vi "PhotonPoseEstimator_Execute.vi"(7 "Configuration":T9, 9 "ReferencePose":T4={"Translation3d"={"X"=0.0, "Y"=0.0, "Z"=0.0}, "Rotation3d"={"Q_quaternion"={"R"=1.0, "V"=[0.0, 0.0, 0.0]}}} {"Translation3d"."Z" format="%14.3f"; "Translation3d"."Y" format="%14.3f"; "Translation3d"."X" format="%14.3f"}, 10 "PIpeline Has \nNew Results":bool, 11 "PipelineResult":T10) -> (0 "TimeStamp_Seconds":dbl, 1 "New Pose Found":bool, 2 "EstimatedPose2d":T1={"TRANSLATION"={"X"=0.0, "Y"=0.0}, "ROTATION"={"VALUE"=0.0, "COS"=1.0, "SIN"=0.0}} {"ROTATION"."SIN" format="%13.4f"; "ROTATION"."COS" format="%13.4f"; "ROTATION"."VALUE" format="%13.4f"; "TRANSLATION"."Y" format="%14.3f"; "TRANSLATION"."X" format="%14.3f"}, 3 "EstimatedPose3d":T4={"Translation3d"={"X"=0.0, "Y"=0.0, "Z"=0.0}, "Rotation3d"={"Q_quaternion"={"R"=1.0, "V"=[0.0, 0.0, 0.0]}}} {"Translation3d"."Z" format="%14.3f"; "Translation3d"."Y" format="%14.3f"; "Translation3d"."X" format="%14.3f"}, 4 "Strategy Used":T8, 5 "PhotonEstimatedRobotPose":T11={"EstimatedPose"={"Translation3d"={"X"=0.0, "Y"=0.0, "Z"=0.0}, "Rotation3d"={"Q_quaternion"={"R"=1.0, "V"=[0.0, 0.0, 0.0]}}}, "TimeStamp_Seconds"=0.0, "targetsUsed"=[], "Strategy"=enum."LOWEST_AMBIGUITY"} {"targetsUsed"."AltCameraToTarget"."TRANSLATION3D"."Z" format="%14.3f"; "targetsUsed"."AltCameraToTarget"."TRANSLATION3D"."Y" format="%14.3f"; "targetsUsed"."AltCameraToTarget"."TRANSLATION3D"."X" format="%14.3f"; "targetsUsed"."BestCameraToTarget"."TRANSLATION3D"."Z" format="%14.3f"; "targetsUsed"."BestCameraToTarget"."TRANSLATION3D"."Y" format="%14.3f"; "targetsUsed"."BestCameraToTarget"."TRANSLATION3D"."X" format="%14.3f"; "EstimatedPose"."Translation3d"."Z" format="%14.3f"; "EstimatedPose"."Translation3d"."Y" format="%14.3f"; "EstimatedPose"."Translation3d"."X" format="%14.3f"}, 6 "out PhotonPoseEstimator":T15)   [LabVIEW 2019, in "PhotonVisionLib.lvlib"]
doc: "Provided data from polling a camera, update the estimated position of the robot. Returns empty if there are no cameras set or no targets were found from the cameras. \n\nInputs:\n -- PhotonPoseEstimator -- data cluster -- Data guiding how the position determination is done.\n -- PipelineResults -- data cluster -- Data provided from PhotonCamera_GetLatestResults.\n -- HasResults -- boolean - TRUE if targets have been identified in the Pipeline results. This can be provided by PhotonCamera_GetLatestResults.\n\nOutputs:\n - EstimatedPose3d - Pose3d - Estimated 3d position. Only value if NewPoseFound = TRUE\n - EstimatedPose2d - Pose2d - Estimated 2d position. Only value if NewPoseFound = TRUE\n - NewPoseFound -- boolean -- A new position has been determined.\n - TimeStampe - double - Target timestamp (seconds)\n - StrategyUsed -- enum -- The strategy used to determine the pose.\n - PhotonEstimatedRobotPose -- data cluster -- Complete estimated robot position and timestamp data cluster\n -- PhotonPoseEstimator -- data cluster -- Updated data cluster."
uses:
  PhotonVisionLib.lvlib
  Ref/PhotonPoseEstimator_REF.ctl
  TypeDef/PhotonPoseEstimatorType.ctl
  <vilib>/Rock Robotics/WPI/ThirdParty/JAS_Junk/TrajLib/TypeDef/POSE3D.ctl
  <vilib>/Rock Robotics/WPI/ThirdParty/JAS_Junk/TrajLib/TypeDef/TRANSLATION3D.ctl
  <vilib>/Rock Robotics/WPI/ThirdParty/JAS_Junk/TrajLib/TypeDef/ROTATION3D.ctl
  <vilib>/Rock Robotics/WPI/ThirdParty/JAS_Junk/TrajLib/TypeDef/QUATERNION.ctl
  <vilib>/Rock Robotics/WPI/ThirdParty/JAS_Junk/TrajLib/TypeDef/AprilTagFieldLayout.ctl
  <vilib>/Rock Robotics/WPI/ThirdParty/JAS_Junk/TrajLib/TypeDef/AprilTag.ctl
  <vilib>/Rock Robotics/WPI/ThirdParty/JAS_Junk/TrajLib/Enum/AprilTagFieldLayoutOrignPosition_ENUM.ctl
  Enum/PhotonPoseStrategy_ENUM.ctl
  <vilib>/Rock Robotics/WPI/ThirdParty/JAS_Junk/TrajLib/TypeDef/TRANSFORM3D.ctl
  TypeDef/PhotonTargetModel.ctl
  TypeDef/PhotonEstimatedRobotPoseType.ctl
  TypeDef/PhotonTrackedTargetType.ctl
  TypeDef/TargetCornerType.ctl
  Ref/PhotonPipelineResult_REF.ctl
  TypeDef/PhotonPipelineResultType.ctl
  TypeDef/PhotonMultiTargetPNPResultType.ctl
  TypeDef/PhotonPNPResultType.ctl
  TypeDef/PhotonPoseEstimator_Configuration.ctl
  <vilib>/Rock Robotics/WPI/ThirdParty/JAS_Junk/TrajLib/TypeDef/POSE2D.ctl
  <vilib>/Rock Robotics/WPI/ThirdParty/JAS_Junk/TrajLib/TypeDef/TRANSLATION2D.ctl
  <vilib>/Rock Robotics/WPI/ThirdParty/JAS_Junk/TrajLib/TypeDef/ROTATION2D.ctl
  <vilib>/Rock Robotics/WPI/ThirdParty/JAS_Junk/TrajLib/VI/Transform3d_GetTranslation3d.vi
  <vilib>/Rock Robotics/WPI/ThirdParty/JAS_Junk/TrajLib/VI/Transform3d_GetRotation3d.vi
  <vilib>/Rock Robotics/WPI/ThirdParty/JAS_Junk/TrajLib/VI/Rotation3d_Equals.vi
  <vilib>/Rock Robotics/WPI/ThirdParty/JAS_Junk/TrajLib/VI/Translation3d_Equals.vi
  <vilib>/Rock Robotics/WPI/ThirdParty/JAS_Junk/TrajLib/VI/AprilTagFieldLayout_New2022.vi
  <vilib>/Rock Robotics/WPI/ThirdParty/JAS_Junk/TrajLib/VI/AprilTagFieldLayout_New2023.vi
  <vilib>/Rock Robotics/WPI/ThirdParty/JAS_Junk/TrajLib/VI/AprilTagFieldLayout_New2024.vi
  PhotonPoseEstimator_Update_All.vi
  <vilib>/Rock Robotics/WPI/ThirdParty/JAS_Junk/TrajLib/VI/Pose3d_getTranslation3d.vi
  <vilib>/Rock Robotics/WPI/ThirdParty/JAS_Junk/TrajLib/VI/Pose3d_getRotation3d.vi
  <vilib>/Rock Robotics/WPI/ThirdParty/JAS_Junk/TrajLib/VI/Translation3d_ToTranslation2d.vi
  <vilib>/Rock Robotics/WPI/ThirdParty/JAS_Junk/TrajLib/VI/Rotation3d_ToRotation2d.vi
  <vilib>/Rock Robotics/WPI/ThirdParty/JAS_Junk/TrajLib/Pose2d_New_TRRO.vi
  <vilib>/Rock Robotics/WPI/ThirdParty/JAS_Junk/TrajLib/VI/Rotation3d_GetQuaterion.vi
  <vilib>/Rock Robotics/WPI/ThirdParty/JAS_Junk/TrajLib/VI/Quaternion_Equals.vi
  <vilib>/Rock Robotics/WPI/ThirdParty/JAS_Junk/TrajLib/VI/AprilTagFieldLayout_New.vi
  <vilib>/Rock Robotics/WPI/ThirdParty/JAS_Junk/TrajLib/VI/Translation3d_Create.vi
  <vilib>/Rock Robotics/WPI/ThirdParty/JAS_Junk/TrajLib/VI/Quaternion_New.vi
  <vilib>/Rock Robotics/WPI/ThirdParty/JAS_Junk/TrajLib/VI/Pose3d_New_Trans3dRot3d.vi
  <vilib>/Rock Robotics/WPI/ThirdParty/JAS_Junk/TrajLib/VI/Rotation3d_Create_Quaternion.vi
  <vilib>/Rock Robotics/WPI/ThirdParty/JAS_Junk/TrajLib/VI/AprilTag_New.vi
  PhotonPoseEstimator_GetEmptyPose.vi
  PhotonPoseEstimator_lowestAmbiguityStrategy.vi
  PhotonPoseEstimator_closestToCameraHeightStrategy.vi
  PhotonPoseEstimator_closestToReferencePoseStrategy.vi
  PhotonPoseEstimator_GetReferencePose.vi
  PhotonPoseEstimator_GetLastPose.vi
  PhotonPoseEstimator_averageBestTargetsStrategy.vi
  PhotonPoseEstimator_multiTagOnCoprocStrategy.vi
  PhotonPoseEstimator_SetPoseCacheTimeout.vi
  PhotonPipelineResult_GetTimeStampSecs.vi
  PhotonPoseEstimator_GetStrategy.vi
  PhotonPoseEstimator_GetPoseCacheTimeout.vi
  <vilib>/Rock Robotics/WPI/ThirdParty/JAS_Junk/TrajLib/Translation2d_Create.vi
  <vilib>/Rock Robotics/WPI/ThirdParty/JAS_Junk/TrajLib/Rotation2d_CreateAngle.vi
  <vilib>/Rock Robotics/WPI/ThirdParty/JAS_Junk/TrajLib/VI/Rotation3d_GetXYZ.vi
  <vilib>/Rock Robotics/WPI/ThirdParty/JAS_Junk/TrajLib/VI/Quaternion_Get_Vect.vi
  <vilib>/Rock Robotics/WPI/ThirdParty/JAS_Junk/TrajLib/VI/Quaternion_Get_W.vi
  <vilib>/Rock Robotics/WPI/ThirdParty/JAS_Junk/TrajLib/VI/AprilTag_GetAll.vi
  <vilib>/Rock Robotics/WPI/ThirdParty/JAS_Junk/TrajLib/VI/Quaternion_Normalize.vi
  <vilib>/Rock Robotics/WPI/ThirdParty/JAS_Junk/TrajLib/VI/Rotation3d_Create_AxisAngle.vi
  <vilib>/Rock Robotics/WPI/ThirdParty/JAS_Junk/TrajLib/VI/Pose3d_New.vi
  PhotonPipelineResult_HasTargets.vi
  PhotonPipelineResult_GetTargets.vi
  PhotonTrackedTarget_GetPoseAmbiguity.vi
  PhotonTrackedTarget_GetFiducialId.vi
  PhotonPoseEstimator_GetFieldTags.vi
  <vilib>/Rock Robotics/WPI/ThirdParty/JAS_Junk/TrajLib/VI/AprilTagFieldLayout_GetTagPose.vi
  <vilib>/Rock Robotics/WPI/ThirdParty/JAS_Junk/TrajLib/VI/Pose3d_TransformBy.vi
  PhotonTrackedTarget_GetBestCameraToTarget.vi
  <vilib>/Rock Robotics/WPI/ThirdParty/JAS_Junk/TrajLib/VI/Transform3d_Inverse.vi
  PhotonPoseEstimator_GetRobotToCameraTransform.vi
  PhotonPoseEstimator_GetHighestAmbiguity.vi
  PhotonEstimatedRobotPose_New.vi
  PhotonPoseEstimator_closestToCameraHeightStrategy_calc.vi
  PhotonTrackedTarget_GetAltCameraToTarget.vi
  PhotonPoseEstimator_closestToReferencePoseStrategy_calc.vi
  PhotonPoseEstimator_averageBestTargetsStrategy_calc.vi
  <vilib>/Rock Robotics/WPI/ThirdParty/JAS_Junk/TrajLib/VI/Rotation3d_Plus.vi
  <vilib>/Rock Robotics/WPI/ThirdParty/JAS_Junk/TrajLib/VI/Translation3d_Plus.vi
  <vilib>/Rock Robotics/WPI/ThirdParty/JAS_Junk/TrajLib/VI/Translation3d_Times.vi
  <vilib>/Rock Robotics/WPI/ThirdParty/JAS_Junk/TrajLib/VI/Rotation3d_Times.vi
  <vilib>/Rock Robotics/WPI/ThirdParty/JAS_Junk/TrajLib/VI/Rotation3d_Create_Default.vi
  <vilib>/Rock Robotics/WPI/ThirdParty/JAS_Junk/TrajLib/VI/Translation3d_Create_Default.vi
  <vilib>/Rock Robotics/WPI/ThirdParty/JAS_Junk/TrajLib/VI/Pose3d_New_Default.vi
  <vilib>/Rock Robotics/WPI/ThirdParty/JAS_Junk/TrajLib/VI/Pose3d_Plus.vi
  <vilib>/Rock Robotics/WPI/ThirdParty/JAS_Junk/TrajLib/VI/Pose3d_RelativeTo.vi
  <vilib>/Rock Robotics/WPI/ThirdParty/JAS_Junk/TrajLib/VI/AprilTagFieldLayout_GetOriginPosition.vi
  PhotonPipelineResult_GetMultiTagResult.vi
  <vilib>/Rock Robotics/WPI/ThirdParty/JAS_Junk/TrajLib/VI/Quaternion_Get_All.vi
  <vilib>/Rock Robotics/WPI/ThirdParty/JAS_Junk/TrajLib/VI/Quaternion_New_Default.vi
  <vilib>/Rock Robotics/WPI/ThirdParty/JAS_Junk/TrajLib/VI/Vector_Norm.vi
  <vilib>/Rock Robotics/WPI/ThirdParty/JAS_Junk/TrajLib/VecBuilder_ArrayBy1Fill.vi
  PhotonPipelineResult_GetTargetCount.vi
  <vilib>/Rock Robotics/WPI/ThirdParty/JAS_Junk/TrajLib/VI/Translation3d_RotateBy.vi
  <vilib>/Rock Robotics/WPI/ThirdParty/JAS_Junk/TrajLib/Transform2d_Create_TransRot.vi
  <vilib>/Rock Robotics/WPI/ThirdParty/JAS_Junk/TrajLib/VI/Transform3d_Create_Trans3dRot3d.vi
  <vilib>/Rock Robotics/WPI/ThirdParty/JAS_Junk/TrajLib/VI/Rotation3d_UnaryMinus.vi
  <vilib>/Rock Robotics/WPI/ThirdParty/JAS_Junk/TrajLib/VI/Translation3d_UnaryMinus.vi
  <vilib>/Rock Robotics/WPI/ThirdParty/JAS_Junk/TrajLib/VI/Transform3d_GetXYZ.vi
  <vilib>/Rock Robotics/WPI/ThirdParty/JAS_Junk/TrajLib/VI/Pose3d_getXYZ.vi
  PhotonPoseEstimator_CalcDifference.vi
  <vilib>/Rock Robotics/WPI/ThirdParty/JAS_Junk/TrajLib/VI/Rotation3d_RotateBy.vi
  <vilib>/Rock Robotics/WPI/ThirdParty/JAS_Junk/TrajLib/VI/Translation3d_GetXYZ.vi
  <vilib>/Rock Robotics/WPI/ThirdParty/JAS_Junk/TrajLib/VI/Transform3d_Create_Pose3dPose3d.vi
  <vilib>/Rock Robotics/WPI/ThirdParty/JAS_Junk/TrajLib/MatBuilder_Create.vi
  <vilib>/Rock Robotics/WPI/ThirdParty/JAS_Junk/TrajLib/VI/Quaternion_Times.vi
  <vilib>/Rock Robotics/WPI/ThirdParty/JAS_Junk/TrajLib/VI/Quaternion_Inverse.vi
  <vilib>/Rock Robotics/WPI/ThirdParty/JAS_Junk/TrajLib/VI/Translation3d_GetDistance.vi
  <vilib>/Rock Robotics/WPI/ThirdParty/JAS_Junk/TrajLib/VI/Translation3d_Minus.vi
  <vilib>/Rock Robotics/WPI/ThirdParty/JAS_Junk/TrajLib/VI/Rotation3d_Minus.vi
  <vilib>/Rock Robotics/WPI/ThirdParty/JAS_Junk/TrajLib/Trajectory_Library.lvlib
  Ref/PhotonPoseEstimator_Configuration_REF.ctl
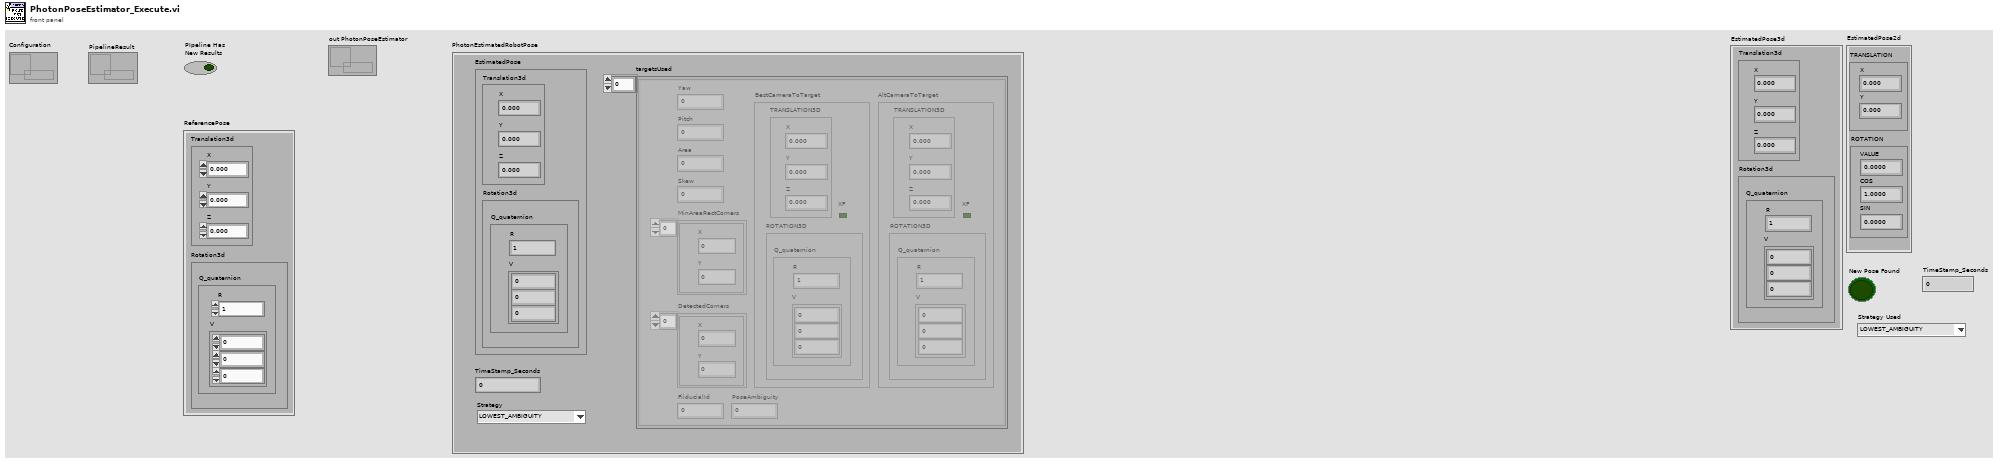
[diagram p1: front panel]
types:
  T1 = typedef "Trajectory_Library.lvlib/POSE2D.ctl" = cluster{"TRANSLATION":T2, "ROTATION":T3}
  T2 = typedef "Trajectory_Library.lvlib/TRANSLATION2D.ctl" = cluster{"X":dbl, "Y":dbl}
  T3 = typedef "Trajectory_Library.lvlib/ROTATION2D.ctl" = cluster{"VALUE":dbl, "COS":dbl, "SIN":dbl}
  T4 = typedef "Trajectory_Library.lvlib/POSE3D.ctl" = cluster{"Translation3d":T5, "Rotation3d":T6}
  T5 = typedef "Trajectory_Library.lvlib/TRANSLATION3D.ctl" = cluster{"X":dbl, "Y":dbl, "Z":dbl}
  T6 = typedef "Trajectory_Library.lvlib/ROTATION3D.ctl" = cluster{"Q_quaternion":T7}
  T7 = typedef "Trajectory_Library.lvlib/QUATERNION.ctl" = cluster{"R":dbl, "V":dbl[]}
  T8 = typedef "PhotonVisionLib.lvlib/PhotonPoseStrategy_ENUM.ctl" = enum16{"LOWEST_AMBIGUITY", "CLOSEST_TO_CAMERA_HEIGHT", "CLOSEST_TO_REFERENCE_POSE", "CLOSEST_TO_LAST_POSE", "AVERAGE_BEST_TARGETS", "MULTI_TAG_PNP_ON_COPROCESSOR", "MULTI_TAG_PNP_ON_RIO"}
  T9 = typedef "PhotonVisionLib.lvlib/PhotonPoseEstimator_Configuration_REF.ctl" = refnum<data-value>
  T10 = typedef "PhotonVisionLib.lvlib/PhotonPipelineResult_REF.ctl" = refnum<data-value>
  T11 = typedef "PhotonVisionLib.lvlib/PhotonEstimatedRobotPoseType.ctl" = cluster{"EstimatedPose":T4, "TimeStamp_Seconds":dbl, "targetsUsed":T12[], "Strategy":T8}
  T12 = typedef "PhotonVisionLib.lvlib/PhotonTrackedTargetType.ctl" = cluster{"Yaw":dbl, "Pitch":dbl, "Area":dbl, "Skew":dbl, "MinAreaRectCorners":T13[], "BestCameraToTarget":T14, "FiiducialId":i32, "AltCameraToTarget":T14, "PoseAmbiguity":dbl, "DetectedCorners":T13[]}
  T13 = typedef "PhotonVisionLib.lvlib/TargetCornerType.ctl" = cluster{"X":dbl, "Y":dbl}
  T14 = typedef "Trajectory_Library.lvlib/TRANSFORM3D.ctl" = cluster{"TRANSLATION3D":T5, "ROTATION3D":T6, "XF":bool}
  T15 = typedef "PhotonVisionLib.lvlib/PhotonPoseEstimator_REF.ctl" = refnum<data-value>
  T16 = typedef "PhotonVisionLib.lvlib/PhotonPoseEstimator_Configuration.ctl" = cluster{"Primary Strategy":T8, "Camera":string, "Initial Pose":T4, "HighestAmbiguity":dbl, "Use Custom Field":bool, "Custom AprilTag Field":T17, "RobotToCamera":T14, "FallBack Strategy":T8, "BaseNTName":string, "AprilTagField":enum16{"2022 Rapid React", "2023 Charged Up", "2024 Crescendo"}}
  T17 = typedef "Trajectory_Library.lvlib/AprilTagFieldLayout.ctl" = cluster{"AprilTagMap":map{i32, T18}, "FieldLength":dbl, "FieldWidth":dbl, "OriginPosition ":T19, "OriginPose3d":T4}
  T18 = typedef "Trajectory_Library.lvlib/AprilTag.ctl" = cluster{"ID":i32, "POSE3D":T4}
  T19 = typedef "Trajectory_Library.lvlib/AprilTagFieldLayoutOrignPosition_ENUM.ctl" = enum16{"kBlueAllianceWallRightSide,", "kRedAllianceWallRightSide,"}
  T20 = enum16{"2022 Rapid React", "2023 Charged Up", "2024 Crescendo"}
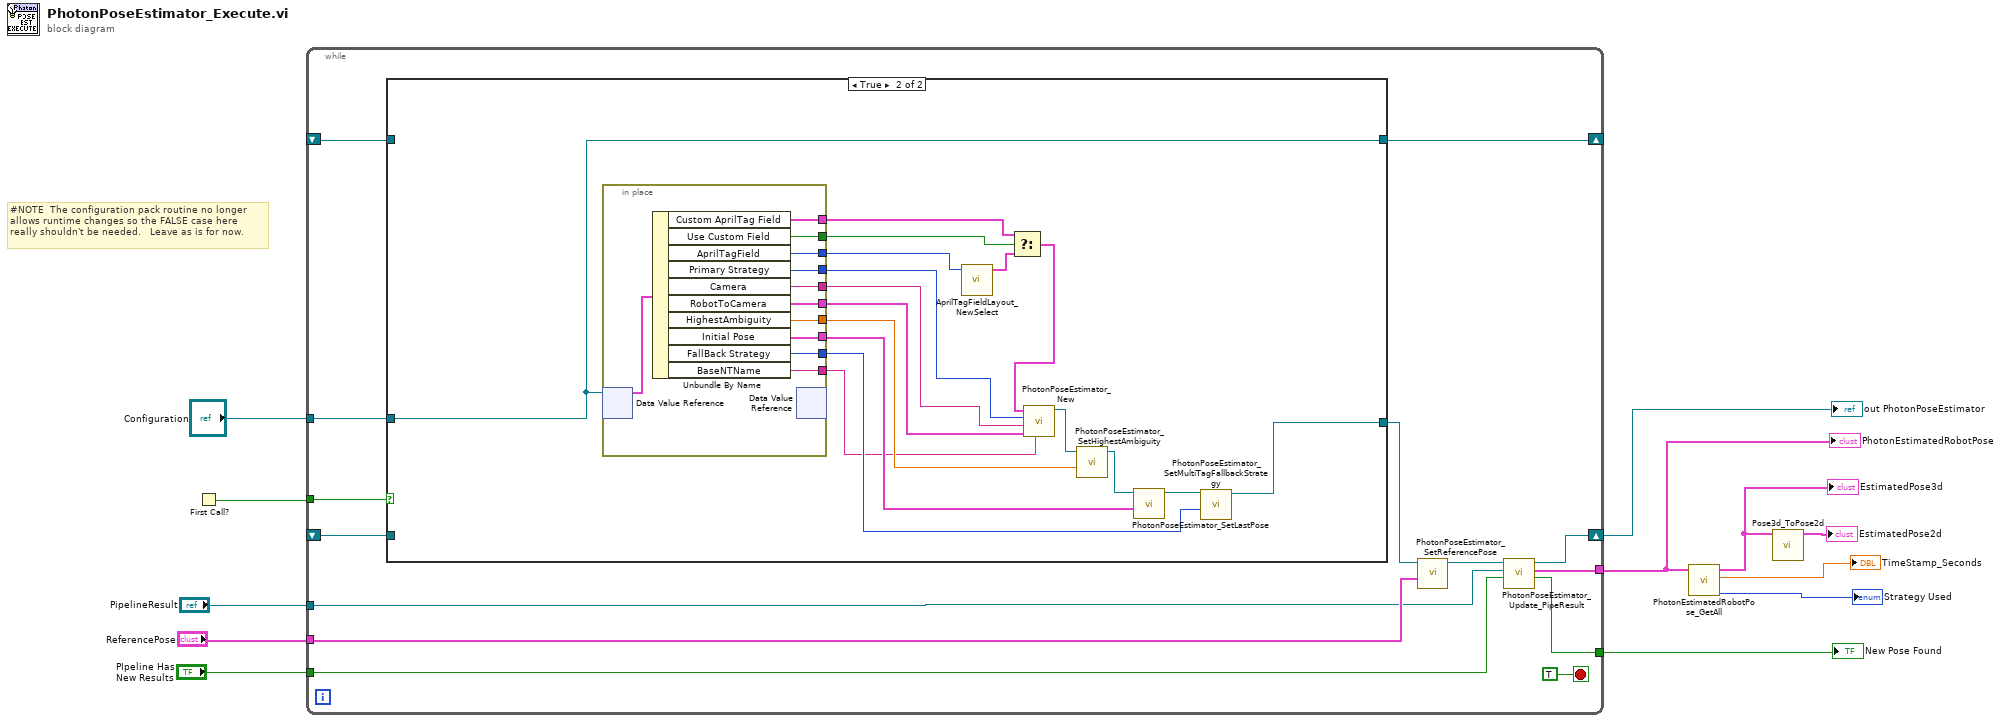
[diagram p0: block diagram]
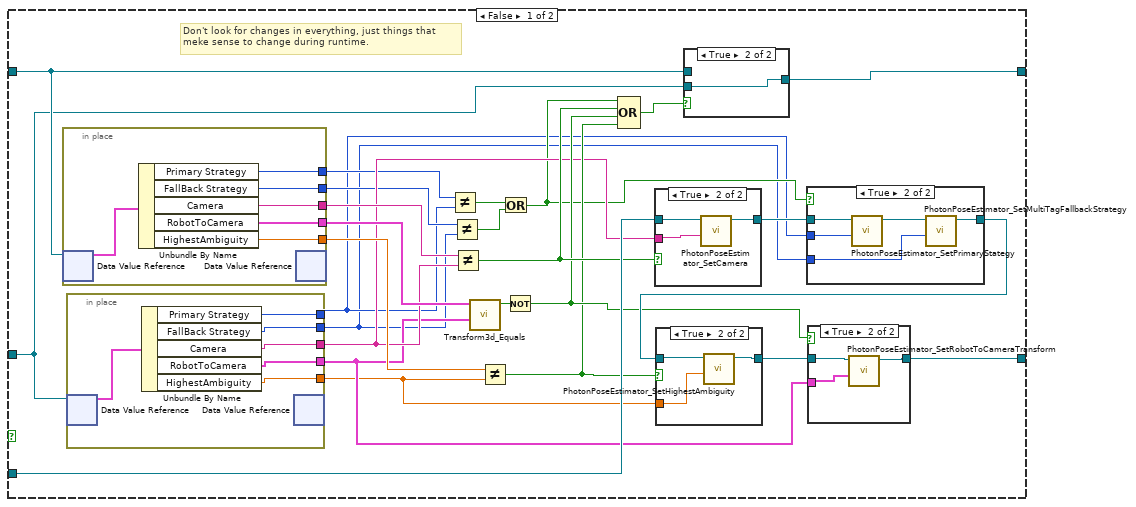
[diagram p2: hidden frame]
diagram:
  # "#NOTE  The configuration pack routine no longer\nallows runtime changes so the FALSE case here\nreally shouldn't be needed.   Leave as is for now."
  n1 = First Call?() -> (First Call?: T/F=w12:bool)
  n2 = while {
    tunnel: w12 -> [w13]
    tunnel: "PipelineResult" -> [w22]
    shift-right: [w20] -> w8
    shift-left: _ -> [w25]
    tunnel: "ReferencePose" -> [w24]
    tunnel: "PIpeline Has \nNew Results" -> [w21]
    tunnel: [w19] -> w5
    tunnel: [w17] -> w7
    tunnel: "Configuration" -> [w15]
    shift-right: [w16] -> _
    shift-left: _ -> [w14]
    stop <- TRUE stop-if-true
    n3 = case shown="True" w13 {
      tunnel: [w29 w88] -> w18
      tunnel: w25 -> [w48 _]
      tunnel: w15 -> [w27 w85]
      tunnel: [w49 w85] -> w16
      tunnel: w14 -> [w28 _]
      frame False {
        # "Don't look for changes in everything, just things that\nmeke sense to change during runtime."
        n4 = in-place {
          in-place-border: [w64] -> w52
          in-place-border: [w63] -> w45
          in-place-border: [w62] -> w41
          in-place-border: [w61] -> w33
          in-place-border: [w60] -> w32
          n5 = in-place-dvr #1(w28) -> (w59:T16)  [unwired: 1 out]
          n6 = Unbundle By Name(w59) -> ("Primary Strategy"=w61:T8, "FallBack Strategy"=w60:T8, "Camera"=w63:string, "RobotToCamera"=w62:T14, "HighestAmbiguity"=w64:dbl)
          n7 = in-place-dvr #1() -> ()  [unwired: 1 in, 2 out]
        }
        n8 = in-place {
          in-place-border: [w58] -> w39
          in-place-border: [w57] -> w38
          in-place-border: [w56] -> w37
          in-place-border: [w55] -> w31
          in-place-border: [w54] -> w30
          n9 = in-place-dvr #2(w27) -> (w53:T16)  [unwired: 1 out]
          n10 = Unbundle By Name(w53) -> ("Primary Strategy"=w55:T8, "FallBack Strategy"=w54:T8, "Camera"=w58:string, "RobotToCamera"=w57:T14, "HighestAmbiguity"=w56:dbl)
          n11 = in-place-dvr #2() -> ()  [unwired: 1 in, 2 out]
        }
        n12 = Not Equal?(x=w33, y=w31) -> (x != y?=w35:bool)
        n13 = Not Equal?(x=w32, y=w30) -> (x != y?=w34:bool)
        n14 = Not Equal?(x=w45, y=w39) -> (x != y?=w46:bool)
        n15 = call <vilib>:"Transform3d_Equals.vi"("otherTransform3d"=w38, "inTransform3d"=w41) -> ("Equals"=w51:bool)  [unwired: 9 in]
        n16 = Not Equal?(x=w52, y=w37) -> (x != y?=w40:bool)
        n17 = Or(x=w35, y=w34) -> (x .or. y?=w36:bool)
        n18 = Not(x=w51) -> (.not. x?=w42:bool)
        n19 = Compound Arithmetic op=OR(w36, w46, w42, w40) -> (w50:bool)
        n20 = case shown="True" w46 {
          tunnel: w48 -> [w81 w84]
          tunnel: [w81 w83] -> w47
          tunnel: w39 -> [_ w82]
          frame False {
          }
          frame True {
            n21 = call "PhotonPoseEstimator_SetCamera.vi"("Camera"=w82, "PhotonPoseEstimator"=w84) -> ("out PhotonPoseEstimator"=w83:T15)  [unwired: 9 in]
          }
        }
        n22 = case shown="True" w50 {
          tunnel: w27 -> [_ w80]
          tunnel: w28 -> [w79 _]
          tunnel: [w79 w80] -> w49
          frame False {
          }
          frame True {
          }
        }
        n23 = case shown="True" w36 {
          tunnel: w47 -> [w73 w78]
          tunnel: w31 -> [_ w77]
          tunnel: [w73 w75] -> w43
          tunnel: w30 -> [_ w74]
          frame False {
          }
          frame True {
            n24 = call "PhotonPoseEstimator_SetPrimaryStategy.vi"("PrimaryStrategy"=w77, "PhotonPoseEstimator"=w78) -> ("out PhotonPoseEstimator"=w76:T15)  [unwired: 9 in]
            n25 = call "PhotonPoseEstimator_SetMultiTagFallbackStrategy.vi"("FallBack Strategy"=w74, "PhotonPoseEstimator"=w76) -> ("out PhotonPoseEstimator"=w75:T15)  [unwired: 9 in]
          }
        }
        n26 = case shown="True" w40 {
          tunnel: w43 -> [w69 w72]
          tunnel: [w69 w71] -> w44
          tunnel: w37 -> [_ w70]
          frame False {
          }
          frame True {
            n27 = call "PhotonPoseEstimator_SetHighestAmbiguity.vi"("HighestAmbiguity"=w70, "PhotonPoseEstimator"=w72) -> ("out PhotonPoseEstimator"=w71:T15)  [unwired: 9 in]
          }
        }
        n28 = case shown="True" w42 {
          tunnel: w44 -> [w65 w68]
          tunnel: [w65 w67] -> w29
          tunnel: w38 -> [_ w66]
          frame False {
          }
          frame True {
            n29 = call "PhotonPoseEstimator_SetRobotToCameraTransform.vi"("RobotToCameraTransform3d"=w66, "PhotonPoseEstimator"=w68) -> ("out PhotonPoseEstimator"=w67:T15)  [unwired: 9 in]
          }
        }
      }
      frame True {
        n30 = in-place {
          in-place-border: [w112] -> w97
          in-place-border: [w111] -> w96
          in-place-border: [w110] -> w95
          in-place-border: [w109] -> w94
          in-place-border: [w108] -> w93
          in-place-border: [w107] -> w92
          in-place-border: [w106] -> w91
          in-place-border: [w105] -> w90
          in-place-border: [w104] -> w87
          in-place-border: [w103] -> w86
          n31 = in-place-dvr #3(w85) -> (w102:T16)  [unwired: 1 out]
          n32 = Unbundle By Name(w102) -> ("Custom AprilTag Field"=w112:T17, "Use Custom Field"=w111:bool, "AprilTagField"=w110:T20, "Primary Strategy"=w109:T8, "Camera"=w108:string, "RobotToCamera"=w107:T14, "HighestAmbiguity"=w106:dbl, "Initial Pose"=w105:T4, "FallBack Strategy"=w104:T8, "BaseNTName"=w103:string)
          n33 = in-place-dvr #3() -> ()  [unwired: 1 in, 2 out]
        }
        n34 = call <vilib>:"AprilTagFieldLayout_NewSelect.vi"("AprilTagField"=w95) -> ("AprilTagFieldLayout"=w99:T17)  [unwired: 10 in]
        n35 = Select(t=w97, s=w96, f=w99) -> (s? t:f=w98:T17)
        n36 = call "PhotonPoseEstimator_New.vi"("BaseNTName"=w86, "RobotToCamera"=w92, "Camera"=w93, "Strategy"=w94, "AprilTagFieldLayout"=w98) -> ("PhotonPoseEstimator"=w101:T15)  [unwired: 6 in]
        n37 = call "PhotonPoseEstimator_SetHighestAmbiguity.vi"("HighestAmbiguity"=w91, "PhotonPoseEstimator"=w101) -> ("out PhotonPoseEstimator"=w100:T15)  [unwired: 9 in]
        n38 = call "PhotonPoseEstimator_SetLastPose.vi"("LastPose"=w90, "PhotonPoseEstimator"=w100) -> ("out PhotonPoseEstimator"=w89:T15)  [unwired: 9 in]
        n39 = call "PhotonPoseEstimator_SetMultiTagFallbackStrategy.vi"("FallBack Strategy"=w87, "PhotonPoseEstimator"=w89) -> ("out PhotonPoseEstimator"=w88:T15)  [unwired: 9 in]
      }
    }
    n40 = call "PhotonPoseEstimator_SetReferencePose.vi"("ReferencePose"=w24, "PhotonPoseEstimator"=w18) -> ("out PhotonPoseEstimator"=w23:T15)  [unwired: 9 in]
    n41 = call "PhotonPoseEstimator_Update_PipeResult.vi"("Has Results"=w21, "PipelineResult"=w22, "PhotonPoseEstimator"=w23) -> ("Pos Found"=w17:bool, "PhotonEstimatedRobotPose"=w19:T11, "out PhotonPoseEstimator"=w20:T15)  [unwired: 6 in]
  }
  "out PhotonPoseEstimator" <- w8
  "PhotonEstimatedRobotPose" <- w5
  "New Pose Found" <- w7
  n42 = call "PhotonEstimatedRobotPose_GetAll.vi"("PhotonEstimatedRobotPose"=w5) -> ("Strategy"=→"Strategy Used":T8, "TimeStamp_Seconds"=→"TimeStamp_Seconds":dbl, "EstimatedPose"=w3:T4)  [unwired: 7 in, 1 out]
  "EstimatedPose3d" <- w3
  n43 = call <vilib>:"Pose3d_ToPose2d.vi"("in Pose3d"=w3) -> ("out Pose2d"=→"EstimatedPose2d":T1)  [unwired: 10 in]
